vi "convertEOL.vi"(2 "Convert EOL? (TRUE)":bool=TRUE, 3 "string":string) -> (1 "string out":string)   [LabVIEW 2011, in "EasyXMLTest.lvclass"]
uses:
  EasyXMLTest.lvclass
  <userlib>/_OpenG.lib/string/string.llb/Convert EOLs (String)__ogtk.vi
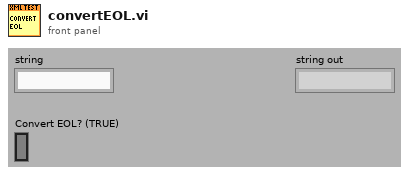
[diagram p1: front panel]
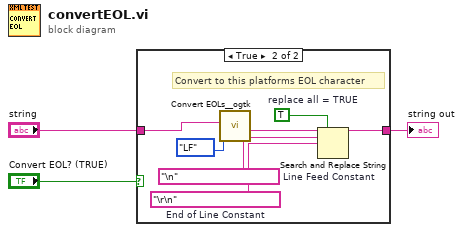
[diagram p0: block diagram]
diagram:
  n1 = case shown="True" "Convert EOL? (TRUE)" {
    tunnel: "string" -> [w4 w11]
    tunnel: [w4 w5] -> w2
    frame False {
    }
    frame True {
      w6 = TRUE  # replace all = TRUE
      w8 = "\r\n"  # End of Line Constant
      w9 = "\n"  # Line Feed Constant
      # "Convert to this platforms EOL character"
      n2 = call-poly <userlib>:"Convert EOLs__ogtk.vi"("Convert to:"=enum16{"CR", "LF", "CRLF"}."LF", "String in"=w11) -> ("String out"=w7:string)  [unwired: 9 in]
      n3 = Search and Replace String(replace all?=w6, input string=w7, search string=w9, replace string=w8) -> (result string=w5:string)  [unwired: 4 in, 3 out]
    }
  }
  "string out" <- w2
